vi "Gif.Main No Read.vi"(0 "bin-string":string, 9 "bgcolor":u32(colorbox)=16777226, 11 "error in (no error)":errorcluster, 12 "image index":i32) -> (6 "time":u32[](array[numeric]), 8 "images out":picture[](array[picture]), 13 "image data":T1, 14 "image size":cluster{"Width":u32, "Height":u32}, 15 "error out":errorcluster)   [LabVIEW 2015]
doc: "This VI reads all images from a gif file.\nCurrently it can only read from version 89a.\nInterlaced images are not taken into account.\n\nThe outputs are an array of all delay times, an array of all images, the image size and an error cluster.\n\nVersion 01.01\nMike Schröder"
uses:
  <vilib>/picture/picture.llb/imagedata.ctl
panel:
  out "color table":u32[](array[colorbox])
  out "Version":string
  out "Signature":string
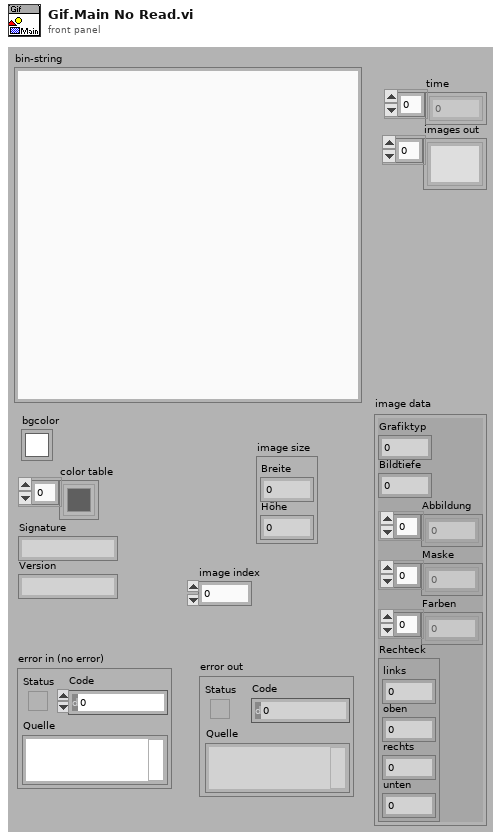
[diagram p1: front panel]
types:
  T1 = typedef "imagedata.ctl" = cluster{"image type":i32, "image depth":i32, "image":u8[], "mask":u8[], "colors":u32[], "Rectangle":cluster{"left":i16, "top":i16, "right":i16, "bottom":i16}}
  T2 = typedef "Gif.LogicalScreenDescriptior.ctl" = cluster{"Logical Screen Width":u16, "Logical Screen Height":u16, "Global Color Table Flag":u8, "Color Resolution":u8, "Sort Flag":u8, "Size of Global Color Table":u8, "Background Color Index":u8, "Pixel Aspect Ratio":u8}
  T3 = typedef "Gif.GraphicControlExtension.ctl" = cluster{"Reserved":u8, "Disposal Method":u8, "User Input Flag":u8, "Transparent Color Flag":u8, "Delay Time":u16, "Transparent Color Index":u8}
  T4 = typedef "Gif.ImageDescriptor.ctl" = cluster{"Image Left Position":u16, "Image Top Position":u16, "Image Width":u16, "Image Height":u16, "Local Color Table Flag":u8, "Interlace Flag":u8, "Sort Flag":u8, "Reserved":u8, "Size Of Local Color Table":u8}
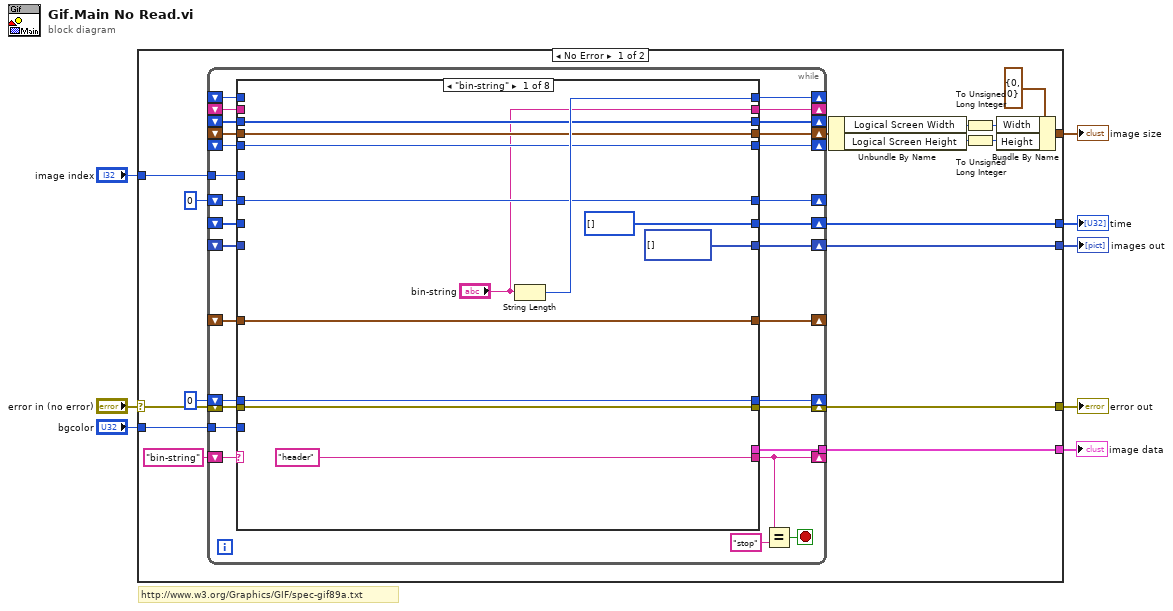
[diagram p0: block diagram]
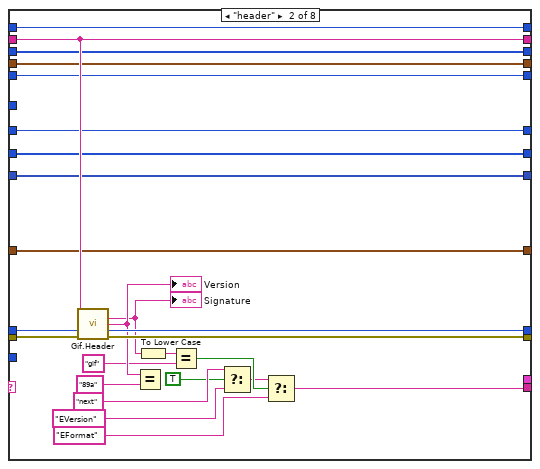
[diagram p2: hidden frame]
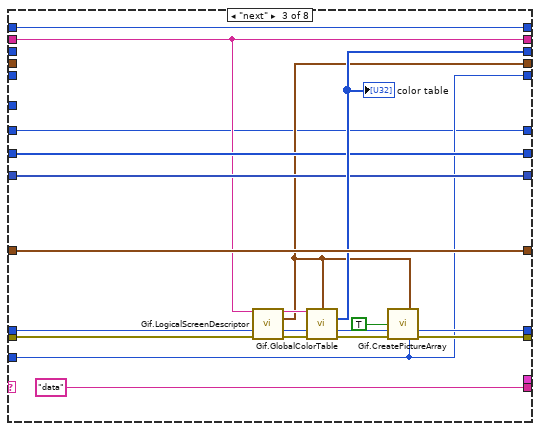
[diagram p3: hidden frame]
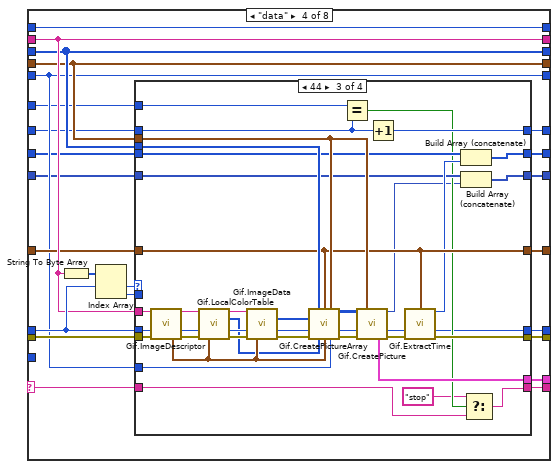
[diagram p4: hidden frame]
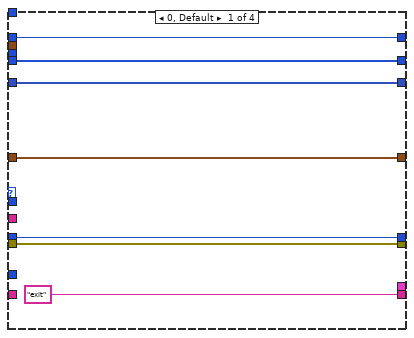
[diagram p5: hidden frame]
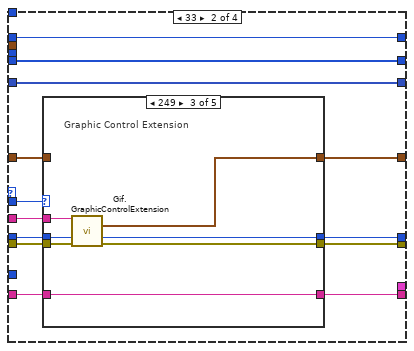
[diagram p6: hidden frame]
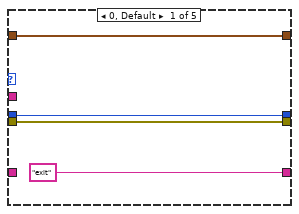
[diagram p7: hidden frame]
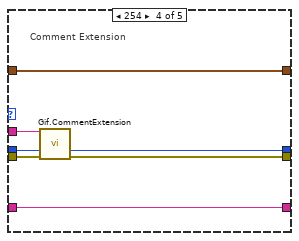
[diagram p9: hidden frame]
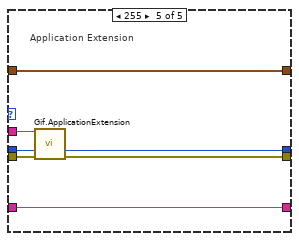
[diagram p10: hidden frame]
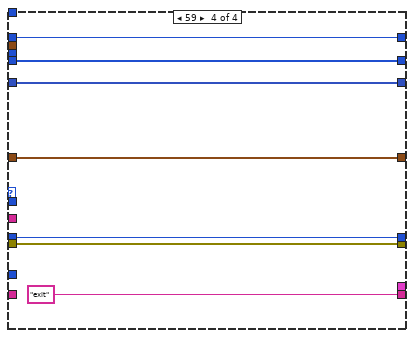
[diagram p11: hidden frame]
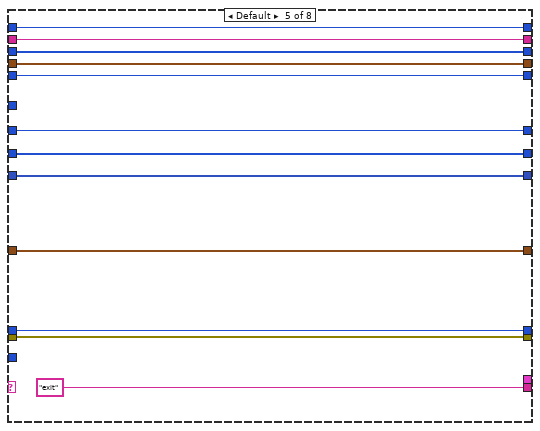
[diagram p12: hidden frame]
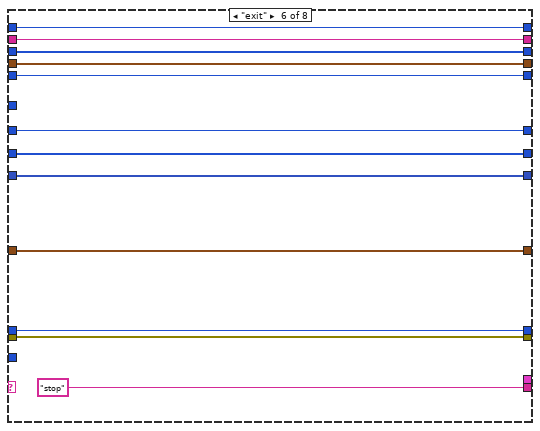
[diagram p13: hidden frame]
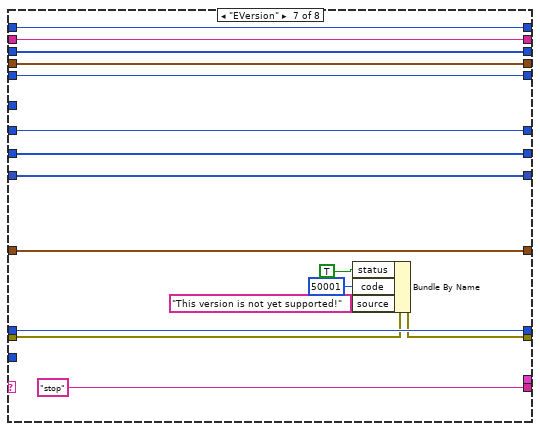
[diagram p14: hidden frame]
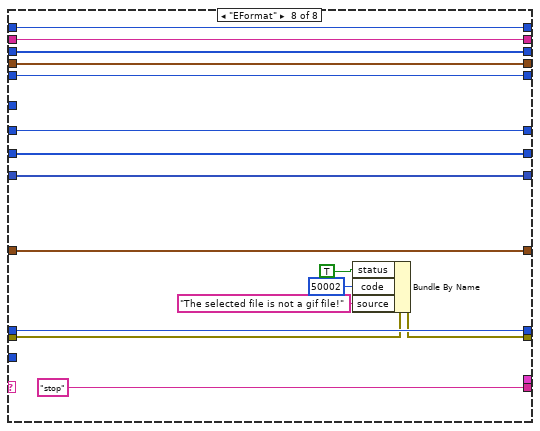
[diagram p15: hidden frame]
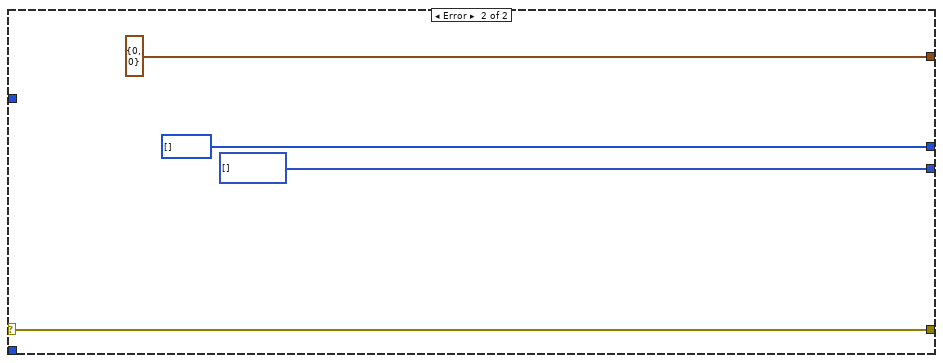
[diagram p16: hidden frame]
diagram:
  # "http://www.w3.org/Graphics/GIF/spec-gif89a.txt"
  n1 = case shown="No Error" "error in (no error)" {
    selector: "error in (no error)" -> [w12 w290]
    tunnel: [w23 u32[] []] -> w8
    tunnel: [w22 picture[] []] -> w1
    tunnel: "bgcolor" -> [w20 _]
    tunnel: [w19 w290] -> w6
    tunnel: [w13 cluster{"Width":u32, "Height":u32} {"Width"=0, "Height"=0} ("Größe des Darstellungsbereichs")] -> w5
    tunnel: "image index" -> [w10 _]
    tunnel: [w9 _] -> w2
    frame No Error {
      n2 = while {
        shift-right: [w45] -> _
        shift-left: "bin-string" -> [w54]
        shift-right: [w53] -> _
        shift-left: _ -> [w51]
        shift-right: [w52] -> _
        shift-left: _ -> [w50]
        shift-right: [w48] -> w19
        shift-left: w12 -> [w49]
        shift-right: [w46] -> _
        shift-left: 0 ("offset (0)") -> [w47]
        shift-right: [w42] -> _
        shift-left: _ -> [w41]
        shift-right: [w40] -> _
        shift-left: _ -> [w39]
        shift-right: [w38] -> w21
        shift-left: _ -> [w37]
        shift-right: [w36] -> _
        shift-left: _ -> [w35]
        shift-right: [w33] -> w23
        shift-left: _ -> [w34]
        shift-right: [w31] -> w22
        shift-left: _ -> [w32]
        tunnel: w20 -> [w30]
        shift-right: [w27] -> _
        shift-left: 0 ("offset (0)") -> [w28]
        tunnel: w10 -> [w26]
        tunnel: [w29] -> w9
        stop <- w43 stop-if-true
        n3 = case shown="\"bin-string\"" w54 {
          selector: w54 -> [_ _ _ w126 _ _ _ _]
          tunnel: [w66 w91 w111 w135 w242 w254 w270 w286] -> w53
          tunnel: ["bin-string" w89 w95 w125 w241 w253 w269 w285] -> w52
          tunnel: w51 -> [_ w91 w111 w135 w242 w254 w270 w286]
          tunnel: w50 -> [_ w89 w95 w125 w241 w253 w269 w285]
          tunnel: ["header" w70 "data" w127 "exit" "stop" "stop" "stop"] -> w45
          tunnel: w49 -> [w56 w90 w94 w130 w239 w251 w260 w276]
          tunnel: [w56 w84 w98 w129 w239 w251 w259 w275] -> w48
          tunnel: w47 -> [w64 w88 w93 w131 w238 w250 w267 w283]
          tunnel: [w64 w83 w100 w128 w238 w250 w267 w283] -> w46
          tunnel: [w63 w82 w105 w124 w237 w249 w266 w282] -> w42
          tunnel: w41 -> [w63 w82 _ w124 w237 w249 w266 w282]
          tunnel: [w62 w87 w109 w123 w236 w248 w265 w281] -> w40
          tunnel: w39 -> [w62 w87 w109 w122 w236 w248 w265 w281]
          tunnel: [w61 w81 w97 w121 w235 w247 w264 w280] -> w38
          tunnel: w37 -> [w61 w81 _ w121 w235 w247 w264 w280]
          tunnel: [w60 w80 w96 w120 w234 w246 w263 w279] -> w36
          tunnel: w35 -> [w60 w80 _ w120 w234 w246 w263 w279]
          tunnel: w34 -> [_ w86 w104 w119 w233 w245 w262 w278]
          tunnel: [u32[] [] w86 w104 w118 w233 w245 w262 w278] -> w33
          tunnel: w32 -> [_ w85 w103 w117 w232 w244 w261 w277]
          tunnel: [picture[] [] w85 w103 w116 w232 w244 w261 w277] -> w31
          tunnel: w30 -> [_ _ w96 _ _ _ _ _]
          tunnel: [_ _ _ w115 _ _ _ _] -> w29
          tunnel: w28 -> [w58 w67 w92 w114 w231 w243 w255 w271]
          tunnel: [w58 w67 w92 w113 w231 w243 w255 w271] -> w27
          tunnel: w26 -> [_ _ _ w112 _ _ _ _]
          frame "bin-string" {
            n4 = String Length(string="bin-string") -> (length=w66:i32)
          }
          frame "header" {
            n5 = call "Gif.Header.vi"("data"=w89, "offset"=w88, "error in (no error)"=w90) -> ("Signature"=w75:string, "Version"=w79:string, "offset out"=w83:i32, "error out"=w84:errorcluster)  [unwired: 1 in, 8 out]
            "Signature" <- w75
            "Version" <- w79
            n6 = Equal?(x=w79, y="89a") -> ()  [unwired: 1 out]
            n7 = To Lower Case(string=w75) -> (all lower case string=w74:string)
            n8 = Equal?(x=w74, y="gif") -> (x = y?=w72:bool)
            n9 = Select(t="next", s=TRUE, f="EVersion") -> (s? t:f=w71:string)
            n10 = Select(t=w71, s=w72, f="EFormat") -> (s? t:f=w70:string)
          }
          frame "next" {
            n11 = call "Gif.LogicalScreenDescriptor.vi"("data"=w95, "offset"=w93, "error in (no error)"=w94) -> ("data out"=w106:string, "Logical Screen Descriptor"=w97:T2, "offset out"=w107:i32, "error out"=w108:errorcluster)  [unwired: 9 out]
            n12 = call "Gif.GlobalColorTable.vi"("data"=w106, "Logical Screen Descriptor"=w97, "offset"=w107, "error in (no error)"=w108) -> ("global color table"=w105:u32[], "offset out"=w101:i32, "error out"=w99:errorcluster)  [unwired: 1 in, 8 out]
            "color table" <- w105
            n13 = call "Gif.CreatePictureArray.vi"("Logical Screen Description"=w97, "init"=TRUE, "offset"=w101, "error in (no error)"=w99, "bgcolor"=w96) -> ("offset out"=w100:i32, "error out"=w98:errorcluster)  [unwired: 5 in, 4 out]
          }
          frame "data" {
            n14 = String To Byte Array(string=w125) -> (unsigned byte array=w134:u8[])
            n15 = Index Array(array=w134, index #1=w131) -> (element #1=w133:u8, element #2=w132:u8)  [unwired: 1 in]
            n16 = case shown="44" w133 {
              tunnel: w132 -> [_ w155 _ _]
              tunnel: w131 -> [w141 w151 w222 w229]
              tunnel: w130 -> [w142 w150 w223 w228]
              tunnel: [w142 w149 w197 w228] -> w129
              tunnel: [w141 w152 w187 w229] -> w128
              tunnel: ["exit" w154 w189 "exit"] -> w127
              tunnel: w126 -> [_ w153 w191 _]
              tunnel: w125 -> [_ w148 w221 _]
              tunnel: w124 -> [_ _ w207 _]
              tunnel: [w139 w147 w205 w227] -> w123
              tunnel: w122 -> [w139 w146 w205 w227]
              tunnel: w121 -> [_ _ w206 _]
              tunnel: w120 -> [_ _ w204 _]
              tunnel: w119 -> [w138 w145 w203 w226]
              tunnel: [w138 w145 w201 w226] -> w118
              tunnel: w117 -> [w137 w144 w200 w225]
              tunnel: [w137 w144 w199 w225] -> w116
              tunnel: [_ _ w195 _] -> w115
              tunnel: w114 -> [w136 w143 w185 w224]
              tunnel: [w136 w143 w193 w224] -> w113
              tunnel: w112 -> [_ _ w194 _]
              frame 0, Default {
              }
              frame 33 {
                n17 = case shown="249" w155 {
                  tunnel: ["exit" w163 w170 w177 w184] -> w154
                  tunnel: w153 -> [_ w163 w170 w177 w184]
                  tunnel: [w158 w162 w166 w174 w182] -> w152
                  tunnel: w151 -> [w158 w162 w168 w175 w183]
                  tunnel: w150 -> [w157 w161 w169 w176 w181]
                  tunnel: [w157 w161 w167 w173 w180] -> w149
                  tunnel: w148 -> [_ _ w165 w172 w179]
                  tunnel: [w156 w160 w164 w171 w178] -> w147
                  tunnel: w146 -> [w156 w160 _ w171 w178]
                  frame 0, Default {
                  }
                  frame 1 {
                  }
                  frame 249 {
                    # "Graphic Control Extension"
                    n18 = call "Gif.GraphicControlExtension.vi"("data"=w165, "offset"=w168, "error in (no error)"=w169) -> ("GraphicControlExtension"=w164:T3, "offset out"=w166:i32, "error out"=w167:errorcluster)  [unwired: 10 out]
                  }
                  frame 254 {
                    # "Comment Extension"
                    n19 = call "Gif.CommentExtension.vi"("data"=w172, "offset"=w175, "error in (no error)"=w176) -> ("offset out"=w174:i32, "error out"=w173:errorcluster)  [unwired: 11 out]
                  }
                  frame 255 {
                    # "Application Extension"
                    n20 = call "Gif.ApplicationExtension.vi"("data"=w179, "offset"=w183, "error in (no error)"=w181) -> ("offset out"=w182:i32, "error out"=w180:errorcluster)  [unwired: 11 out]
                  }
                }
              }
              frame 44 {
                n21 = call "Gif.ImageDescriptor.vi"("data"=w221, "offset"=w222, "error in (no error)"=w223) -> ("data out"=w218:string, "offset out"=w219:i32, "ImageDescriptor"=w209:T4, "error out"=w220:errorcluster)  [unwired: 9 out]
                n22 = call "Gif.LocalColorTable.vi"("data"=w218, "offset"=w219, "error in (no error)"=w220, "ImageDescriptor"=w209) -> ("data out"=w215:string, "local color table"=w208:u32[], "offset out"=w216:i32, "error out"=w217:errorcluster)  [unwired: 5 in, 3 out]
                n23 = call "Gif.ImageData.vi"("data"=w215, "offset"=w216, "error in (no error)"=w217, "ImageDescriptor"=w209) -> ("Index Array"=w213:i32[], "offset out"=w188:i32, "error out"=w214:errorcluster)  [unwired: 1 in, 8 out]
                n24 = call "Gif.CreatePictureArray.vi"("gloal color table"=w207, "GraphicControlExtension"=w205, "Logical Screen Description"=w206, "Index Array"=w213, "offset"=w188, "error in (no error)"=w214, "local color table"=w208, "ImageDescriptor"=w209, "bgcolor"=w204) -> ("image out"=w210:u32[][], "offset out"=w211:i32, "error out"=w212:errorcluster)  [unwired: 1 in, 3 out]
                n25 = Equal?(x=w194, y=w185) -> (x = y?=w192:bool)
                n26 = call "Gif.CreatePicture.vi"("image in"=w210, "Logical Screen Description"=w206, "offset"=w211, "error in (no error)"=w212) -> ("image out"=w186:picture, "offset out"=w196:i32, "graphic data"=w195:T1, "error out"=w198:errorcluster)  [unwired: 8 out]
                n27 = Increment(x=w185) -> (x+1=w193:i32)
                n28 = call "Gif.ExtractTime.vi"("GraphicControlExtension"=w205, "offset"=w196, "error in (no error)"=w198) -> ("time"=w202:u32, "offset out"=w187:i32, "error out"=w197:errorcluster)  [unwired: 10 out]
                n29 = Build Array (concatenate)(w203, w202) -> (w201:u32[])
                n30 = Build Array (concatenate)(w200, w186) -> (w199:picture[])
                n31 = Select(t="stop", s=w192, f=w191) -> (s? t:f=w189:string)
              }
              frame 59 {
              }
            }
          }
          frame Default {
          }
          frame "exit" {
          }
          frame "EVersion" {
            n32 = Bundle By Name(cluster=w260, "status"=TRUE, "code"=50001, "source"="This version is not yet supported!") -> (w259:errorcluster)
          }
          frame "EFormat" {
            n33 = Bundle By Name(cluster=w276, "status"=TRUE, "code"=50002, "source"="The selected file is not a gif file!") -> (w275:errorcluster)
          }
        }
        n34 = Equal?(x=w45, y="stop") -> (x = y?=w43:bool)
      }
      n35 = Unbundle By Name(w21) -> ("Logical Screen Width"=w16:u16, "Logical Screen Height"=w15:u16)
      n36 = To Unsigned Long Integer(number=w16) -> (unsigned 32bit integer=w17:u32)
      n37 = To Unsigned Long Integer(number=w15) -> (unsigned 32bit integer=w18:u32)
      n38 = Bundle By Name(cluster=cluster{"Width":u32, "Height":u32} {"Width"=0, "Height"=0} ("Größe des Darstellungsbereichs"), "Width"=w17, "Height"=w18) -> (w13:cluster{"Width":u32, "Height":u32})
    }
    frame Error {
    }
  }
  "time" <- w8
  "error out" <- w6
  "image size" <- w5
  "image data" <- w2
  "images out" <- w1
